vi "数据存储(子VI).vi"(8 "错误常量 2":errorcluster caption="错误常量", 11 "Array输入":refnum<vi>) -> (0 "错误常量":errorcluster)   [LabVIEW 2016]
uses:
  <vilib>/Utility/file.llb/Write Delimited Spreadsheet (string).vi
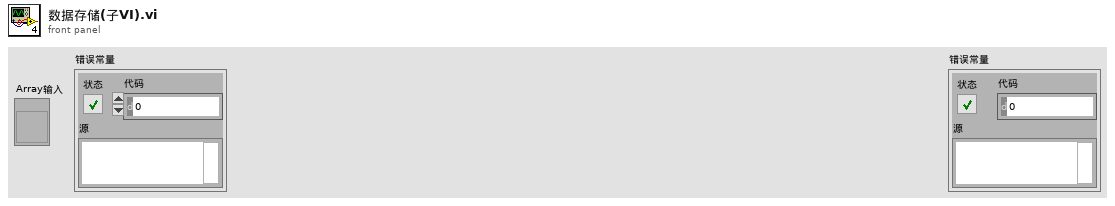
[diagram p1: front panel]
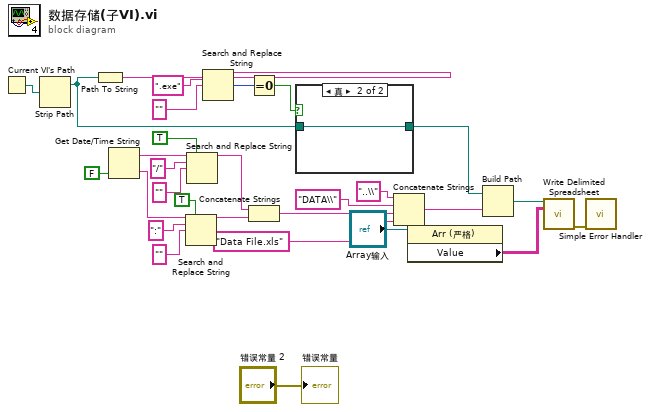
[diagram p0: block diagram]
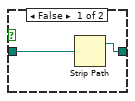
[diagram p2: hidden frame]
diagram:
  n1 = Current VI's Path() -> (path=w16:path)
  n2 = Strip Path(path=w16) -> (stripped path=w23:path)  [unwired: 1 out]
  n3 = Path To String(path=w23) -> (string=w20:string)
  n4 = Get Date/Time String(want seconds? (F)=FALSE ("需要秒？(F)")) -> (date string=w11:string, time string=w14:string)  [unwired: 2 in]
  n5 = Search and Replace String(replace all?=TRUE ("替换全部？(F)"), input string=w14, search string=":" ("搜索字符串"), replace string="" ("替换字符串(\"\")")) -> (result string=w6:string)  [unwired: 4 in, 3 out]
  n6 = Search and Replace String(replace all?=TRUE ("替换全部？(F)"), input string=w11, search string="/" ("搜索字符串"), replace string="" ("替换字符串(\"\")")) -> (result string=w7:string)  [unwired: 4 in, 3 out]
  n7 = Search and Replace String(input string=w20, search string=".exe" ("搜索字符串"), replace string="" ("替换字符串(\"\")")) -> (number of replacements=w26:i32)  [unwired: 5 in, 3 out]
  n8 = Equal To 0?(x=w26) -> (x = 0?=w25:bool)
  n9 = Concatenate Strings(w7, w6) -> (w5:string)
  n10 = case shown="真" w25 {
    tunnel: [w31 w32] -> w24
    tunnel: w23 -> [w30 w32]
    frame False {
      n11 = Strip Path(path=w30) -> (stripped path=w31:path)  [unwired: 1 out]
    }
    frame True {
    }
  }
  n12 = Concatenate Strings("..\\" ("字符串"), "DATA\\" ("字符串"), w5, "Data File.xls" ("name or relative path")) -> (w15:string)
  n13 = property class="Arr (严格)"(reference="Array输入") -> ("Value"=w29:string[][])  [unwired: 1 in, 2 out]
  n14 = Build Path(base path=w24, name or relative path=w15) -> (appended path=w4:path)
  n15 = call-poly <vilib>:"Write Delimited Spreadsheet.vi"("file path (dialog if empty)"=w4, "2D data"=w29) -> ("error out"=w3:errorcluster)  [unwired: 12 in, 1 out]
  n16 = call <vilib>:"Simple Error Handler.vi"("error in (no error)"=w3) -> ()  [unwired: 4 in, 5 out]
  "错误常量" <- "错误常量 2"
